vi "Calc Collapse Bounds.vi"(10 "Panel Height":i16, 11 "Panel Width":i16) -> (3 "Collapsed Bounds":T1)   [LabVIEW 2020, in "PicoG-Processor.lvlib" / "GVIWebProcessorApp.lvclass"]
uses:
  GVIWebProcessorApp.lvclass
  <vilib>/Utility/miscctls.llb/LVRectTypeDef.ctl
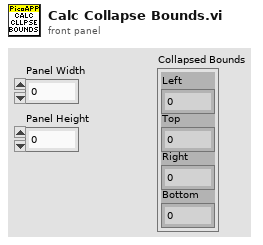
[diagram p1: front panel]
types:
  T1 = typedef "LVRectTypeDef.ctl" = cluster{"Left":i16, "Top":i16, "Right":i16, "Bottom":i16}
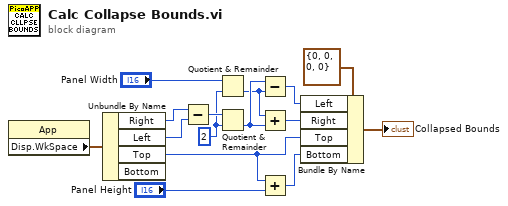
[diagram p0: block diagram]
diagram:
  w10 = i16 2 ("y")
  n1 = property class="App"() -> ("Disp.WkSpace"=w15:T1)  [unwired: 2 in, 2 out]
  n2 = Unbundle By Name(w15) -> ("Right"=w14:i16, "Left"=w13:i16, "Top"=w3:i16)  [unwired: 1 out]
  n3 = Subtract(x=w14, y=w13) -> (x-y=w12:i16)
  n4 = Quotient & Remainder(x="Panel Width", y=w10) -> (floor(x/y)=w8:i16)  [unwired: 1 out]
  n5 = Quotient & Remainder(x=w12, y=w10) -> (floor(x/y)=w9:i16)  [unwired: 1 out]
  n6 = Subtract(x=w9, y=w8) -> (x-y=w4:i16)
  n7 = Add(x=w8, y=w9) -> (x+y=w5:i16)
  n8 = Add(x=w3, y="Panel Height") -> (x+y=w2:i16)
  n9 = Bundle By Name(cluster=T1 {"Left"=0, "Top"=0, "Right"=0, "Bottom"=0} ("input cluster"), "Left"=w4, "Right"=w5, "Top"=w3, "Bottom"=w2) -> (→"Collapsed Bounds":T1)
